vi "nominal_channel_writer.write_batches_from_waveform.vi"(7 "Channel":string, 8 "error in":errorcluster, 9 "Waveform":waveform(dbl), 10 "Data Source RID":string, 11 "Nominal Client in":refnum<class "Nominal Client.lvclass">) -> (0 "error out":errorcluster, 3 "Nominal Client out":refnum<class "Nominal Client.lvclass">)   [LabVIEW 2020, in "Nominal Client.lvclass"]
doc: "Synchronously writes batches of records to a Nominal data source from a LabVIEW Waveform.\n\nThe Attributes of the LabVIEW Waveform will be parsed as tags. <b>note: </b>Only String attributes will be parsed and sent to Nominal Core."
uses:
  Nominal Client.lvclass
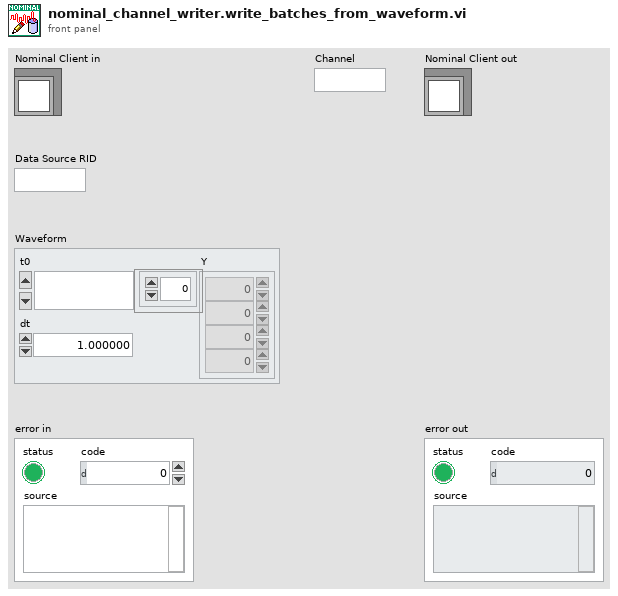
[diagram p1: front panel]
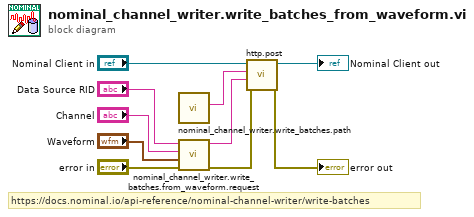
[diagram p0: block diagram]
diagram:
  # "https://docs.nominal.io/api-reference/nominal-channel-writer/write-batches"
  n1 = call "nominal_channel_writer.write_batches.path.vi"() -> ("Path"=w7:string)  [unwired: 11 in]
  n2 = call "nominal_channel_writer.write_batches.from_waveform.request.vi"("error in"="error in", "Waveform"="Waveform", "Channel"="Channel", "Data Source RID"="Data Source RID") -> ("error out"=w5:errorcluster, "Response body"=w6:string)  [unwired: 6 in]
  n3 = call "http.post.vi"("error in"=w5, "Request body"=w6, "Path"=w7, "Nominal Client in"="Nominal Client in") -> ("error out"=→"error out":errorcluster, "Nominal Client out"=→"Nominal Client out":refnum<class "Nominal Client.lvclass">)  [unwired: 4 in, 2 out]
